vi "WM Input-Output Random Seas (math only).vi"(0 "Output Time Series":dbl[](array[numeric]) format="%.2f", 1 "Run":bool, 2 "Start up/Continue":bool, 5 "Sampling Rate":dbl format="%.2f", 7 "Sub Buffer Size":dbl format="%.2f", 9 "Output Task ID In":u32, 11 "Input Task ID In":u32, 12 "error in (no error)":errorcluster, 13 "End":bool) -> (4 "Buffer":dbl[](array[numeric]) format="%.2f", 6 "Experimental Data":dbl[][](array[numeric]) format="%.2f", 8 "Output Task ID Out":u32, 10 "Input Task ID Out":u32, 14 "End Out":bool, 15 "error out":errorcluster)   [LabVIEW 2012]
uses:
  <vilib>/Analysis/1siggen.llb/Ramp Pattern by Samples.vi
  <vilib>/Analysis/NI_AALBase.lvlib
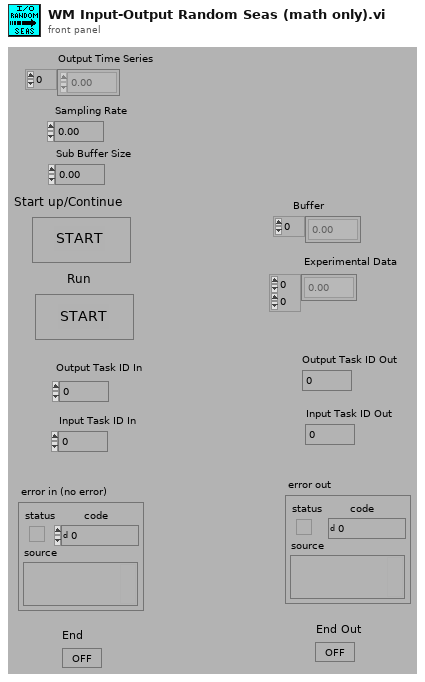
[diagram p1: front panel]
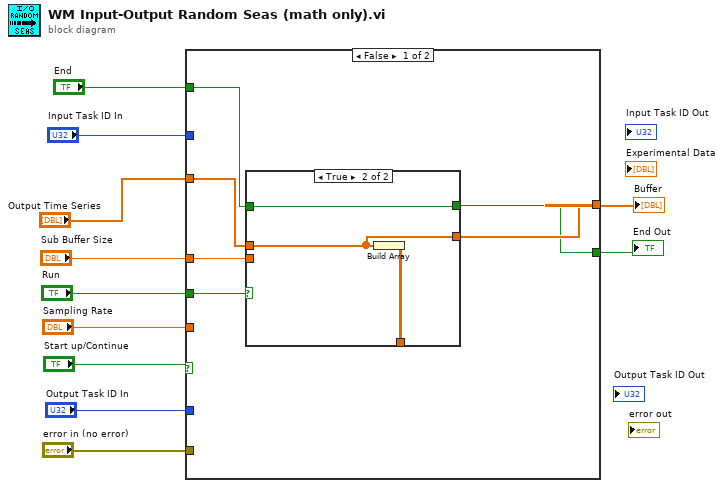
[diagram p0: block diagram]
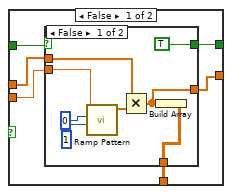
[diagram p2: hidden frame]
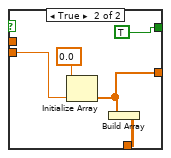
[diagram p3: hidden frame]
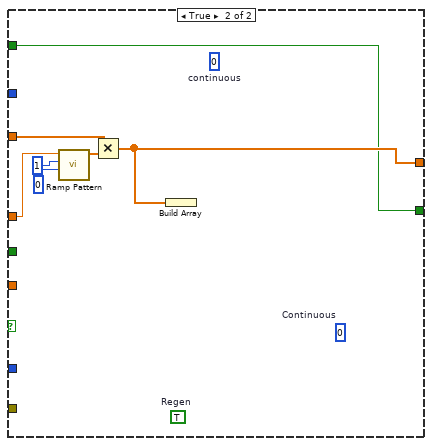
[diagram p4: hidden frame]
diagram:
  n1 = case shown="False" "Start up/Continue" {
    tunnel: "Output Time Series" -> [w17 w43]
    tunnel: "Sub Buffer Size" -> [w14 w41]
    tunnel: [w16 w42] -> w10
    tunnel: "Run" -> [w15 _]
    tunnel: "error in (no error)" -> [_ _]
    tunnel: "Output Task ID In" -> [_ _]
    tunnel: "Sampling Rate" -> [_ _]
    tunnel: "Input Task ID In" -> [_ _]
    tunnel: "End" -> [w13 w40]
    tunnel: [w12 w40] -> w1
    frame False {
      n2 = case shown="True" w15 {
        tunnel: w17 -> [w23 w39]
        tunnel: w14 -> [w22 _]
        tunnel: [w21 w39] -> w16
        tunnel: [w20 w38] -> _
        tunnel: w13 -> [w19 w37]
        tunnel: [w18 w37] -> w12
        frame False {
          n3 = case shown="False" w19 {
            tunnel: w23 -> [w31 _]
            tunnel: w22 -> [w30 w34]
            tunnel: [w29 w36] -> w21
            tunnel: [w28 w35] -> w20
            tunnel: [TRUE TRUE] -> w18
            frame False {
              n4 = call-poly <vilib>:"Ramp Pattern.vi"("start"=i8 1, "end"=i8 0, "samples"=w30) -> ("Ramp Pattern"=w25:dbl[])  [unwired: 7 in, 1 out]
              n5 = Multiply(x=w31, y=w25) -> (x*y=w29:dbl[])
              n6 = Build Array(w29) -> (w28:dbl[][])
            }
            frame True {
              n7 = Initialize Array(0.0 ("Element Data"), w34) -> (w36:dbl[])
              n8 = Build Array(w36) -> (w35:dbl[][])
            }
          }
        }
        frame True {
          n9 = Build Array(w39) -> (w38:dbl[][])
        }
      }
    }
    frame True {
      (unwired) 0  # continuous
      (unwired) TRUE  # Regen
      (unwired) 0  # Continuous
      n10 = call-poly <vilib>:"Ramp Pattern.vi"("start"=i8 0, "end"=i8 1, "samples"=w41) -> ("Ramp Pattern"=w44:dbl[])  [unwired: 7 in, 1 out]
      n11 = Multiply(x=w43, y=w44) -> (x*y=w42:dbl[])
      n12 = Build Array(w42) -> ()  [unwired: 1 out]
    }
  }
  "Buffer" <- w10
  "End Out" <- w1
